vi "mclamp_zero_pipetteCap.vi"(8 "error in (no error)":errorcluster, 10 "Error in":i32, 11 "Multiclamp Handle Out":u32) -> (0 "error out":errorcluster, 2 "slow comp (pF)":dbl, 3 "fast comp (pF)":dbl)   [LabVIEW 2019]
uses:
  patcherBot_software_all/patcherBot_Software/patcherBot/AxMultiClampMsg.dll
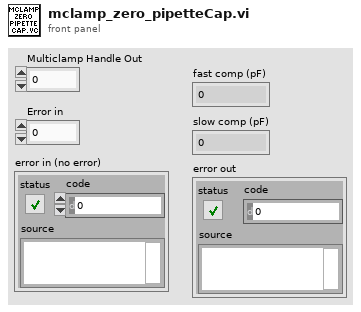
[diagram p1: front panel]
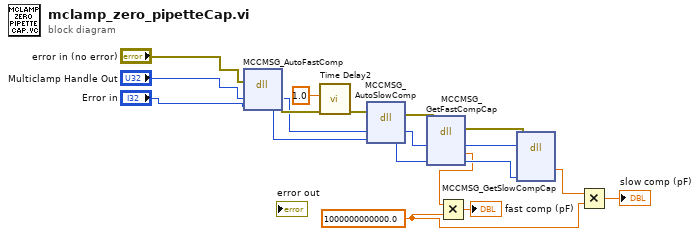
[diagram p0: block diagram]
diagram:
  w4 = 1000000000000.0 ("y")
  n1 = dll-call lib="C:/Users/might/Dropbox (GaTech)/patcherBot_software_all/patcherBot_Software/patcherBot/AxMultiClampMsg.dll" fn="MCCMSG_AutoFastComp"(error in="error in (no error)", "handle"="Multiclamp Handle Out", "error"="Error in") -> (error out=w18:errorcluster, "handle"=w16:u32, "error"=w15:i32)  [unwired: 3 in, 1 out]
  n2 = call "Time Delay2"("error in (no error)"=w18, "Delay Time (s)"=1.0) -> ("error out"=w17:errorcluster)  [unwired: 9 in]
  n3 = dll-call lib="C:/Users/might/Dropbox (GaTech)/patcherBot_software_all/patcherBot_Software/patcherBot/AxMultiClampMsg.dll" fn="MCCMSG_AutoSlowComp"(error in=w17, "handle"=w16, "error"=w15) -> (error out=w14:errorcluster, "handle"=w12:u32, "error"=w11:i32)  [unwired: 3 in, 1 out]
  n4 = dll-call lib="C:/Users/might/Dropbox (GaTech)/patcherBot_software_all/patcherBot_Software/patcherBot/AxMultiClampMsg.dll" fn="MCCMSG_GetFastCompCap"(error in=w14, "handle"=w12, "error"=w11) -> (error out=w13:errorcluster, "handle"=w10:u32, "pdFastCompCap"=w8:dbl, "error"=w9:i32)  [unwired: 4 in, 1 out]
  n5 = Multiply(x=w8, y=w4) -> (x*y=→"fast comp (pF)":dbl)
  n6 = dll-call lib="C:/Users/might/Dropbox (GaTech)/patcherBot_software_all/patcherBot_Software/patcherBot/AxMultiClampMsg.dll" fn="MCCMSG_GetSlowCompCap"(error in=w13, "handle"=w10, "error"=w9) -> ("pdSlowCompCap"=w5:dbl)  [unwired: 6 in, 2 out]
  n7 = Multiply(x=w5, y=w4) -> (x*y=→"slow comp (pF)":dbl)
